vi "Map UUID LIst.vi"(2 "UUIDs":string[](array[string]), 3 "UUID List":string[](array[string])) -> (0 "remapped?":bool, 1 "indices":i32[](array[numeric]))   [LabVIEW 2020]
uses:
  21be96f9-be59-474a-bb47-ce77f5fd0bb0.vi
  8bda544b-0874-47c6-a529-75f039448b35.vi
  Match 1D Array Elements/Match 1D Array Elements - string.vi
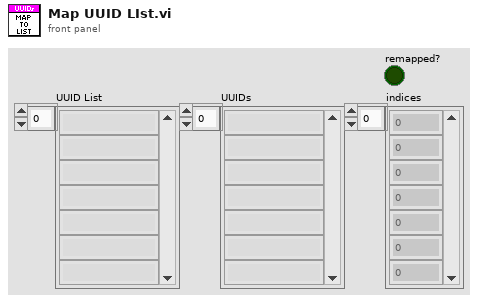
[diagram p1: front panel]
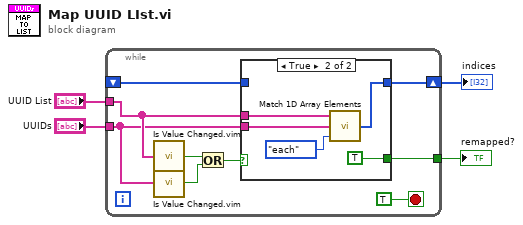
[diagram p0: block diagram]
diagram:
  n1 = while {
    tunnel: "UUID List" -> [w9]
    tunnel: "UUIDs" -> [w7]
    shift-right: [w11] -> w2
    shift-left: _ -> [w10]
    tunnel: [w5] -> w4
    stop <- TRUE stop-if-true
    n2 = call "Is Value Changed.vim"("value"=w9) -> ("changed or first call?"=w8:bool)
    n3 = call "Is Value Changed.vim"("value"=w7) -> ("changed or first call?"=w6:bool)
    n4 = Or(x=w8, y=w6) -> (x .or. y?=w13:bool)
    n5 = case shown="True" w13 {
      tunnel: w9 -> [_ w18]
      tunnel: w7 -> [_ w17]
      tunnel: [w14 w16] -> w11
      tunnel: w10 -> [w14 _]
      tunnel: [_ TRUE] -> w5
      frame False {
      }
      frame True {
        n6 = call-poly "Match 1D Array Elements.vi"("mode (any)"=enum16{"any", "each"}."each", "elements (none)"=w17, "1D Array"=w18) -> ("indices"=w16:i32[])
      }
    }
  }
  "indices" <- w2
  "remapped?" <- w4
